vi "APS start timer.vi"(8 "error in (no error)":errorcluster caption="错误输入（无错误）", 9 "Start":i32, 10 "TrgCh":i32, 11 "Board_ID":i32) -> (0 "error out":errorcluster caption="错误输出", 3 "function return":i32)   [LabVIEW 2011, in "APS168.lvlib"]
doc: "I32 FNTYPE APS_start_timer( I32 Board_ID, I32 TrgCh, I32 Start );"
uses:
  APS168.lvlib
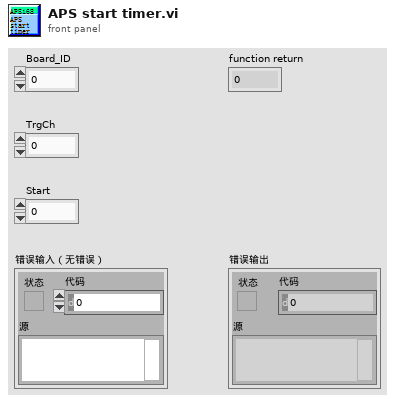
[diagram p1: front panel]
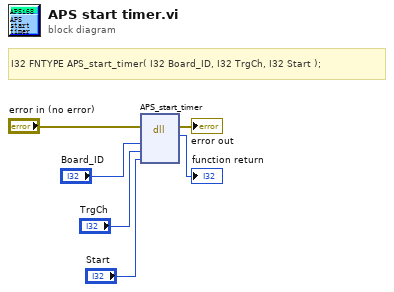
[diagram p0: block diagram]
diagram:
  # "I32 FNTYPE APS_start_timer( I32 Board_ID, I32 TrgCh, I32 Start );"
  n1 = dll-call lib="PTH1Labs E软件ADLINK 204CAPS_1_7_1_LIB line 连续运动204APS168.*" fn="APS_start_timer"(error in="error in (no error)", "Board_ID"="Board_ID", "TrgCh"="TrgCh", "Start"="Start") -> (error out=→"error out":errorcluster, →"function return":i32)  [unwired: 5 in, 1 out]
